vi "Save File Get Max.vi"(8 "Error In":errorcluster, 9 "index (row)":i32=3, 10 "Search Element":string, 11 "Full Data":string[][](array[string])) -> (0 "Error Out":errorcluster, 3 "Max Value":dbl)   [LabVIEW 2016]
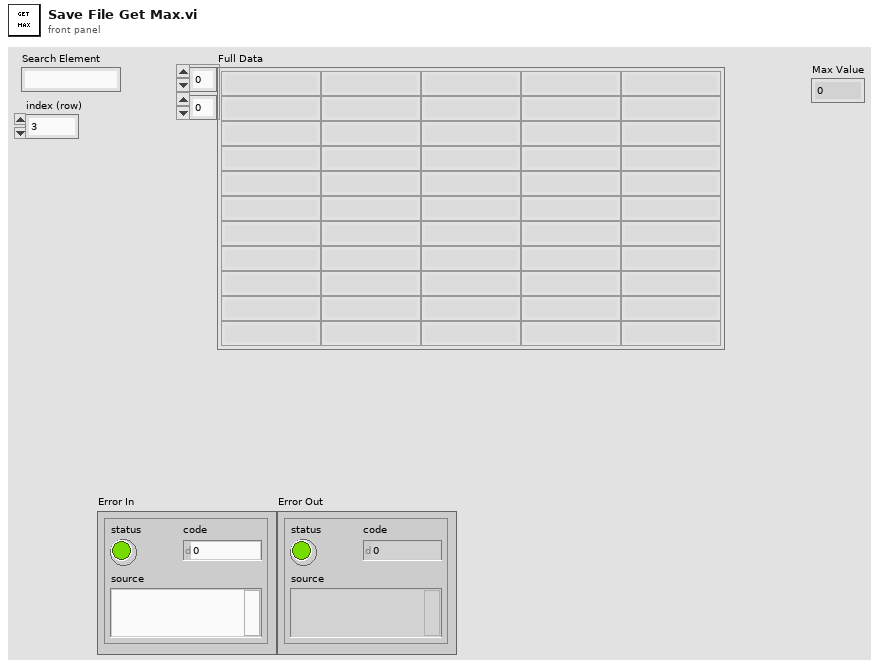
[diagram p1: front panel]
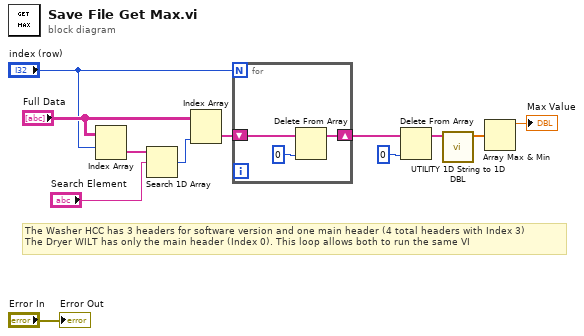
[diagram p0: block diagram]
diagram:
  # "The Washer HCC has 3 headers for software version and one main header (4 total headers with Index 3)\nThe Dryer WILT has only the main header (Index 0). This loop allows both to run the same VI"
  n1 = Index Array(array="Full Data", index (row)="index (row)") -> (element=w6:string[])  [unwired: 1 in]
  n2 = Search 1D Array(1D array=w6, element="Search Element") -> (index of element=w8:i32)  [unwired: 1 in]
  n3 = Index Array(array="Full Data", index (col)=w8) -> (element=w5:string[])  [unwired: 1 in]
  n4 = for {
    N: "index (row)" -> [_]
    shift-right: [w14] -> w3
    shift-left: w5 -> [w15]
    n5 = Delete From Array(array=w15, index=0) -> (array with subset deleted=w14:string[])  [unwired: 1 in, 1 out]
  }
  n6 = Delete From Array(array=w3, index=0) -> (array with subset deleted=w9:string[])  [unwired: 1 in, 1 out]
  n7 = call "UTILITY 1D String to 1D DBL.vi"("Save Data"=w9) -> ("DBL"=w10:dbl[])  [unwired: 10 in]
  n8 = Array Max & Min(array=w10) -> (max value=→"Max Value":dbl)  [unwired: 3 out]
  "Error Out" <- "Error In"
